vi "Poll.vi"(8 "error in (no error)":errorcluster, 10 "Data":variant, 11 "PID Loop in":refnum<class "PID Loop.lvclass">) -> (0 "error out":errorcluster, 3 "PID Loop out":refnum<class "PID Loop.lvclass">)   [LabVIEW 2024, in "PID Loop.lvlib" / "PID Loop.lvclass"]
uses:
  PID Loop.lvclass
  PID Loop.lvclass/PID Loop.ctl
  <vilib>/addons/control/pid/NI_PID_pid.lvlib
  <vilib>/addons/control/pid/pid.llb/PID (DBL).vi
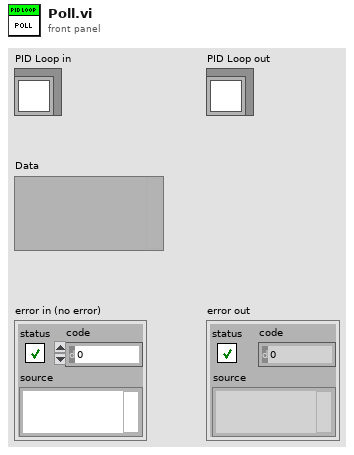
[diagram p1: front panel]
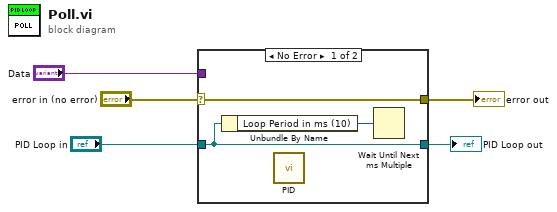
[diagram p0: block diagram]
diagram:
  n1 = case shown="No Error" "error in (no error)" {
    selector: "error in (no error)" -> [w8 w10]
    tunnel: [w8 w10] -> w4
    tunnel: [w7 w9] -> w2
    tunnel: "PID Loop in" -> [w7 w9]
    tunnel: "Data" -> [_ _]
    frame No Error {
      n2 = Unbundle By Name(w7) -> ("Loop Period in ms (10)"=w6:u32)
      n3 = call-poly <vilib>:"PID.vi"() -> ()  [unwired: 10 in, 2 out]
      n4 = Wait Until Next ms Multiple(millisecond multiple=w6) -> ()  [unwired: 1 out]
    }
    frame Error {
    }
  }
  "error out" <- w4
  "PID Loop out" <- w2
